vi "Pat Match Full.vi"(0 "Minimum Match Score":sgl=500.0, 1 "Template File Path":path=path "C:/Users/Admin/Desktop/Main_Module_Assembly/Pattern recognition/templates/color.png", 11 "error in":errorcluster) -> (4 "Matched?":bool, 6 "Score":dbl, 8 "x rel move":dbl, 10 "y rel move":dbl, 15 "error out":errorcluster)   [LabVIEW 2011]
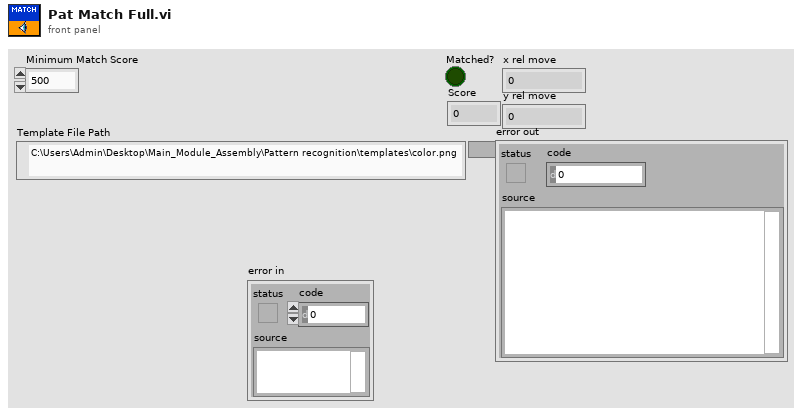
[diagram p1: front panel]
types:
  T1 = typedef "IMAQ Image.ctl" = refnum<image>
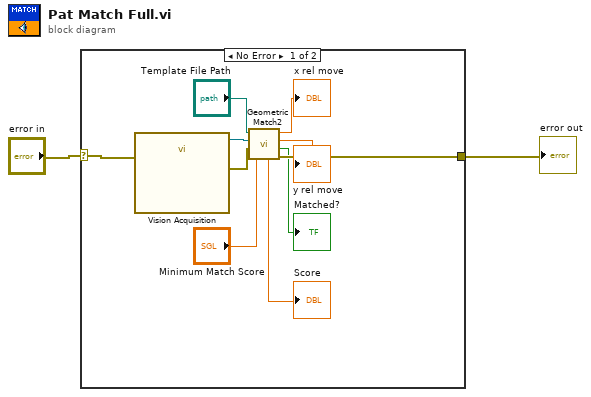
[diagram p0: block diagram]
diagram:
  n1 = case shown="No Error" "error in" {
    selector: "error in" -> [w12 w13]
    tunnel: [w6 w13] -> w1
    frame No Error {
      n2 = call "Vision Acquisition"("error in"=w12) -> ("Image Out"=w10:T1, "error out"=w9:errorcluster)  [unwired: 25 in]
      n3 = call "Geometric Match2.vi"("Template File Path"="Template File Path", "Image Src"=w10, "error in (no error)"=w9, "Minimum Match Score"="Minimum Match Score") -> ("Score"=→"Score":dbl, "x rel move"=→"x rel move":dbl, "y rel move"=→"y rel move":dbl, "Matched?"=→"Matched?":bool, "error out"=w6:errorcluster)
    }
    frame Error {
    }
  }
  "error out" <- w1
